vi "Spartan Builder - Package Built Client.vi"(8 "error in (no error)":errorcluster) -> (0 "error out":errorcluster, 3 "Version":T1 {"Build Date/Time" format="%<%X\n%x>T"})   [LabVIEW 2011]
uses:
  SI.LIB/OGAB Version.ctl
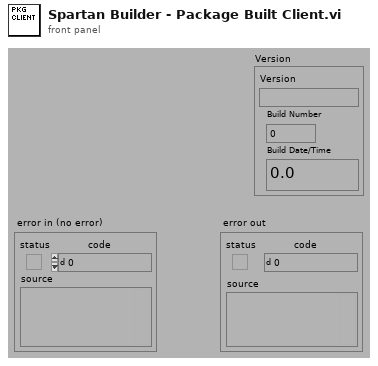
[diagram p1: front panel]
types:
  T1 = typedef "OGAB Version.ctl" = cluster{"Version":string, "Build Number":u32, "Build Date/Time":dbl}
  T2 = enum16{"open", "replace", "create", "open or create", "replace or create", "replace or create with confirmation"}
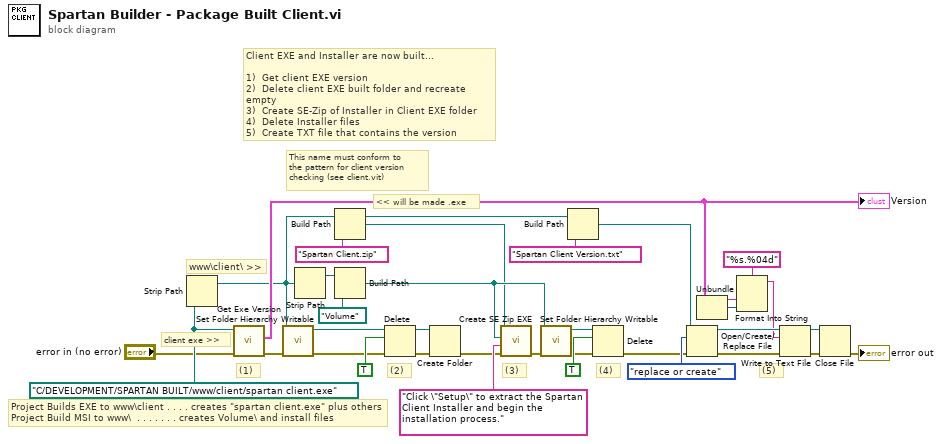
[diagram p0: block diagram]
diagram:
  w32 = path "C:/DEVELOPMENT/SPARTAN BUILT/www/client/spartan client.exe" ("EXE Path (empty - use current)")
  # "(5)"
  # "www\\client\\ >>"
  # "<< will be made .exe"
  # "(4)"
  # "(3)"
  # "(2)"
  # "(1)"
  # "This name must conform to\nthe pattern for client version\nchecking (see client.vit)"
  # "Project Builds EXE to www\\client . . . . creates \"spartan client.exe\" plus others\nProject Build MSI to www\\  . . . . . . . creates Volume\\ and install files"
  # "Client EXE and Installer are now built...\n\n1)  Get client EXE version\n2)  Delete client EXE built folder and recreate empty\n3)  Create SE-Zip of Installer in Client EXE folder\n4)  Delete Installer files\n5)  Create TXT file that contains the version"
  # "client exe >>"
  n1 = Strip Path(path=w32) -> (stripped path=w10:path)  [unwired: 1 out]
  n2 = call "Get Exe Version.vi"("error in (no error)"="error in (no error)", "EXE Path (\"\")"=w32) -> ("error out"=w23:errorcluster, "Version"=w12:T1)  [unwired: 8 out]
  "Version" <- w12
  n3 = call "Set Folder Hierarchy Writable.vi"("error in (no error)"=w23, "Folder Path (empty)"=w10) -> ("error out"=w24:errorcluster, "dup Folder Path"=w22:path)  [unwired: 8 out]
  n4 = Strip Path(path=w10) -> (stripped path=w33:path)  [unwired: 1 out]
  n5 = Build Path(base path=w10, name or relative path="Spartan Client.zip") -> (appended path=w17:path)
  n6 = Build Path(base path=w33, name or relative path=path "Volume") -> (appended path=w18:path)
  n7 = Delete(path (use dialog)=w22, entire hierarchy (F)=TRUE, error in=w24) -> (deleted path=w25:path, error out=w27:errorcluster)  [unwired: 3 out]
  n8 = Create Folder(path (use dialog)=w25, error in=w27) -> (error out=w26:errorcluster)  [unwired: 3 out]
  n9 = call "Create SE Zip EXE.vi"("error in (no error)"=w26, "Setup Dialog Text (\"\")"="Click \"Setup\" to extract the Spartan Client Installer and begin the installation process." ("format string"), "Source File/Directory"=w18, "ZIP Archive Path (empty)"=w17) -> ("error out"=w21:errorcluster)  [unwired: 7 out]
  n10 = call "Set Folder Hierarchy Writable.vi"("error in (no error)"=w21, "Folder Path (empty)"=w18) -> ("error out"=w20:errorcluster, "dup Folder Path"=w19:path)  [unwired: 8 out]
  n11 = Build Path(base path=w10, name or relative path="Spartan Client Version.txt") -> (appended path=w7:path)
  n12 = Delete(path (use dialog)=w19, entire hierarchy (F)=TRUE, error in=w20) -> (error out=w8:errorcluster)  [unwired: 4 out]
  n13 = Open/Create/Replace File(file path (use dialog)=w7, error in=w8, operation (0:open)=T2."replace or create") -> (refnum out=w3:refnum<file>, error out=w6:errorcluster)  [unwired: 3 in, 1 out]
  n14 = Unbundle(w12) -> ("Version"=w14:string, "Build Number"=w13:u32)  [unwired: 1 out]
  n15 = Format Into String(format string="%s.%04d", w14, w13) -> (resulting string=w1:string)  [unwired: 2 in, 1 out]
  n16 = Write to Text File(file (use dialog)=w3, text=w1, error in=w6) -> (refnum out=w2:refnum<file>, error out=w5:errorcluster)  [unwired: 1 in, 1 out]
  n17 = Close File(refnum=w2, error in=w5) -> (error out=→"error out":errorcluster)  [unwired: 1 out]
